vi "ReadScan2_Rf.vi"(8 "error in (no error)":errorcluster, 11 "Data In":T3) -> (0 "error out":errorcluster, 1 "Next State":T2=enum."State1", 2 "States":T1, 3 "Data Out":T3)   [LabVIEW 2014]
doc: "Use this template to build a standard state machine design pattern. Each state executes code and determines which state to transition to. Contrast this design pattern with the User Interface Event Handler pattern, in which code executes in response to user actions. Contrast this design pattern also with the Queued Message Handler pattern, in which each message handling code can queue zero or more new messages.\nNote: This template does not contain the most recent programming guidelines recommended by National Instruments. For a complete, project-based implementation of the Standard State Machine pattern, use the Create Project dialog box instead of this template."
uses:
  controls/Data.ctl
  controls/Wait Scan States.ctl
  controls/State.ctl
  controls/ReadScan1States.ctl
panel:
  # "日期"
  # "機種名稱"
  # "機種代號"
  # "商品條碼"
  # "台"
  # "OK"
  # "NG"
  # "台"
  # "總計"
  # "台"
  # "日期"
  # "機種名稱"
  # "機種代號"
  # "商品條碼"
  # "台"
  # "OK"
  # "NG"
  # "台"
  # "總計"
  # "台"
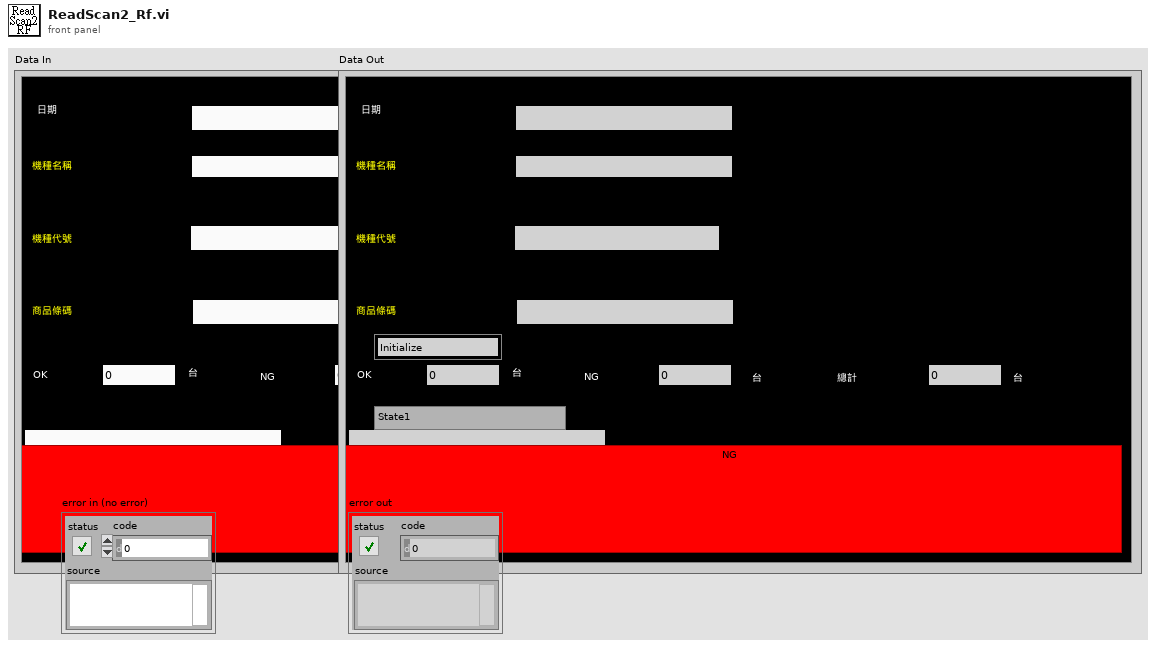
[diagram p1: front panel]
types:
  T1 = typedef "State.ctl" = enum16{"Initialize", "Wait for Scan", "State 1", "State 2", "NG", "NG1", "OK", "OKNG", "Exit"}
  T2 = typedef "Wait Scan States.ctl" = enum16{"Initialize", "State1", "Stop"}
  T3 = typedef "Data.ctl" = cluster{"Date":string, "BarCode1":string, "BarCode2":string, "BarCode3":string, "Message":string, "OK Count":u16, "NG Count":u16, "Total Count":u16, "ModelData":string[][], "OK&NG":bool, "COM1":refnum<visa-resource-name>, "COM2":refnum<visa-resource-name>, "IO":i32, "Time":u32, "TCP":refnum<k5>, "TCP 2":refnum<k5>}
  T4 = typedef "ReadScan1States.ctl" = enum16{"Initialize", "Init2", "Step1", "Step2", "Step3", "Step4", "One", "Two", "Three", "Four", "Five", "End", "Stop"}
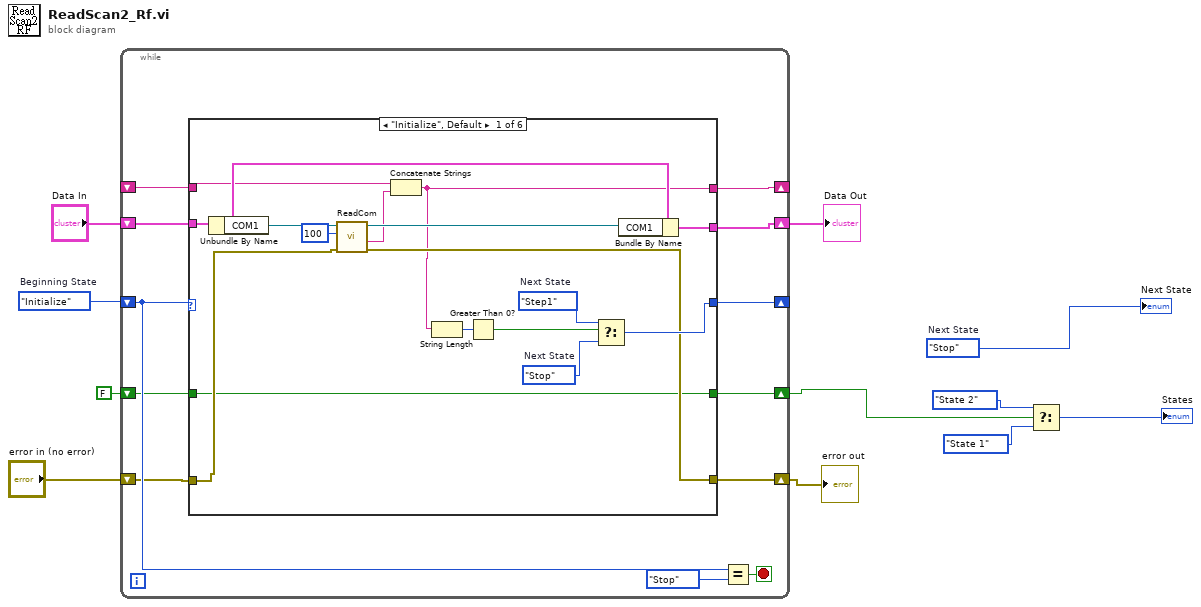
[diagram p0: block diagram]
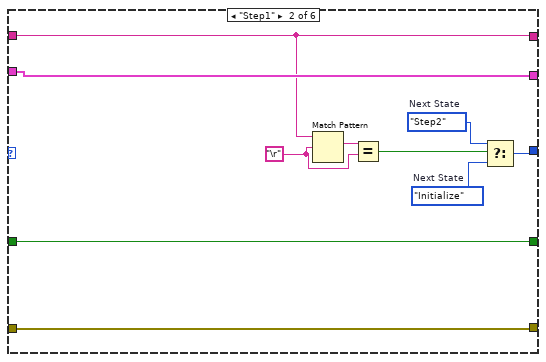
[diagram p2: hidden frame]
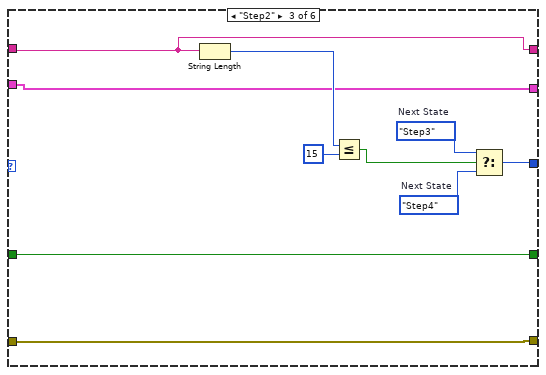
[diagram p3: hidden frame]
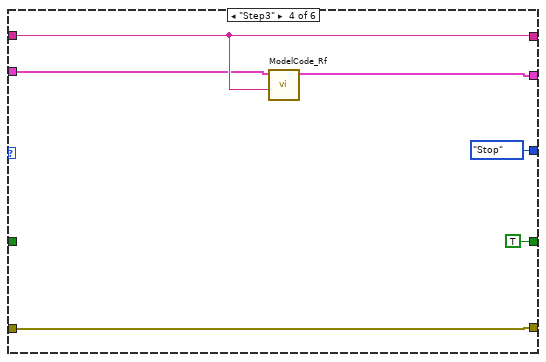
[diagram p4: hidden frame]
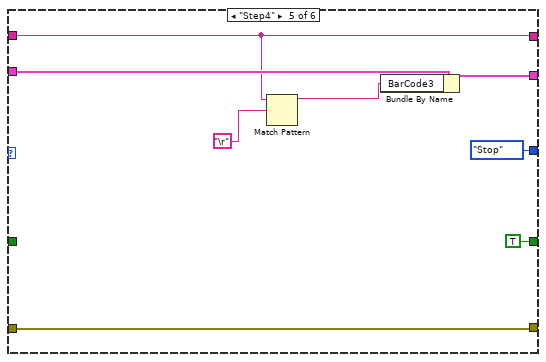
[diagram p5: hidden frame]
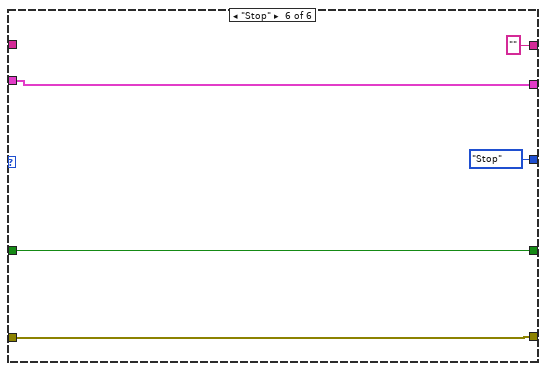
[diagram p6: hidden frame]
diagram:
  w1 = Wait_Scan_States."Stop"  # Next State
  w11 = ReadScan1States."Initialize"  # Beginning State
  n1 = while {
    shift-right: [w20] -> _
    shift-left: w11 -> [w21]
    shift-right: [w15] -> w9
    shift-left: "Data In" -> [w18]
    shift-right: [w14] -> w7
    shift-left: "error in (no error)" -> [w19]
    shift-right: [w16] -> _
    shift-left: _ -> [w17]
    shift-right: [w13] -> w2
    shift-left: FALSE -> [w12]
    stop <- w23 stop-if-true
    n2 = case shown="\"Initialize\", Default" w21 {
      tunnel: [w34 w46 w53 ReadScan1States."Stop" ("Next State") ReadScan1States."Stop" ("Next State") ReadScan1States."Stop" ("Next State")] -> w20
      tunnel: w19 -> [w30 w40 w51 w65 w72 w75]
      tunnel: w18 -> [w33 w49 w57 w61 w70 w76]
      tunnel: w17 -> [w27 w45 w52 w62 w66 _]
      tunnel: [w24 w45 w52 w62 w66 ""] -> w16
      tunnel: [w32 w49 w57 w60 w69 w76] -> w15
      tunnel: [w29 w40 w51 w65 w72 w75] -> w14
      tunnel: [w28 w41 w50 TRUE TRUE w74] -> w13
      tunnel: w12 -> [w28 w41 w50 _ _ w74]
      frame "Initialize", Default {
        w36 = ReadScan1States."Step1"  # Next State
        w35 = ReadScan1States."Stop"  # Next State
        n3 = Unbundle By Name(w33) -> ("COM1"=w39:refnum<visa-resource-name>)
        n4 = call "ReadCom.vi"("error in (no error)"=w30, "delay before read (ms)"=u32 100, "Com In"=w39) -> ("error out"=w29:errorcluster, "Response"=w26:string, "Com Out"=w31:refnum<visa-resource-name>)  [unwired: 5 in, 1 out]
        n5 = Concatenate Strings(w27, w26) -> (w24:string)
        n6 = String Length(string=w24) -> (length=w25:i32)
        n7 = Greater Than 0?(x=w25) -> (x > 0?=w37:bool)
        n8 = Select(t=w36, s=w37, f=w35) -> (s? t:f=w34:T4)
        n9 = Bundle By Name(cluster=w33, "COM1"=w31) -> (w32:T3)
      }
      frame "Step1" {
        w43 = "\r"
        w48 = ReadScan1States."Step2"  # Next State
        w47 = ReadScan1States."Initialize"  # Next State
        n10 = Match Pattern(string=w45, regular expression=w43) -> (match substring=w44:string)  [unwired: 1 in, 3 out]
        n11 = Equal?(x=w44, y=w43) -> (x = y?=w42:bool)
        n12 = Select(t=w48, s=w42, f=w47) -> (s? t:f=w46:T4)
      }
      frame "Step2" {
        w56 = ReadScan1States."Step3"  # Next State
        w55 = ReadScan1States."Step4"  # Next State
        n13 = String Length(string=w52) -> (length=w59:i32)
        n14 = Less Or Equal?(x=w59, y=15) -> (x <= y?=w54:bool)
        n15 = Select(t=w56, s=w54, f=w55) -> (s? t:f=w53:T4)
      }
      frame "Step3" {
        n16 = call "ModelCode_Rf.vi"("BarCode"=w62, "Data In"=w61) -> ("Data Out"=w60:T3)  [unwired: 8 in, 1 out]
      }
      frame "Step4" {
        n17 = Match Pattern(string=w66, regular expression="\r") -> (before substring=w68:string)  [unwired: 1 in, 3 out]
        n18 = Bundle By Name(cluster=w70, "BarCode3"=w68) -> (w69:T3)
      }
      frame "Stop" {
      }
    }
    n19 = Equal?(x=w21, y=ReadScan1States."Stop" ("States")) -> (x = y?=w23:bool)
  }
  "Data Out" <- w9
  "error out" <- w7
  n20 = Select(t=State."State 2" ("States"), s=w2, f=State."State 1" ("States")) -> (s? t:f=→"States":T1)
  "Next State" <- w1
